vi "ConfigureDlg.vi"(8 "error in (no error)":errorcluster, 11 "PmuBase in":refnum<class "SensorBase.lvclass">) -> (0 "error out":errorcluster, 2 "Changed":bool, 3 "PmuBase out":refnum<class "SensorBase.lvclass">)   [LabVIEW 2014, in "SensorPlugins.lvlib" / "SensorBase.lvclass"]
uses:
  SensorBase.lvclass
panel:
  in  "btnDone":bool
  # "No configurable parameters for this Sensor plugin"
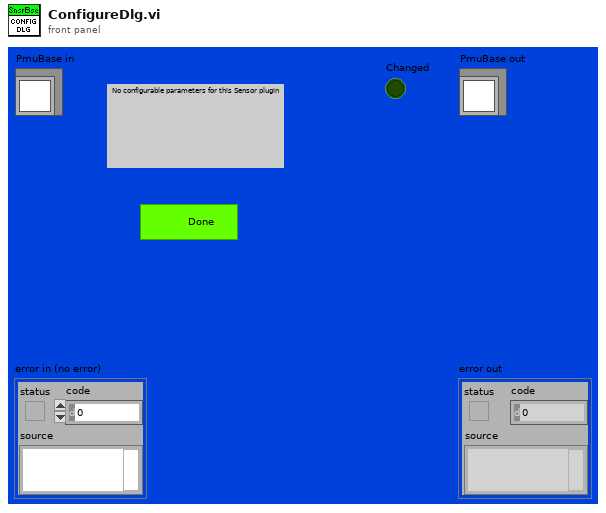
[diagram p1: front panel]
types:
  T1 = enum32{"Invalid", "Standard", "Closed", "Hidden", "Minimized", "Maximized"}
  T2 = enum32{"Invalid", "Default", "Floating", "Floating/Auto-Hide", "Modal"}
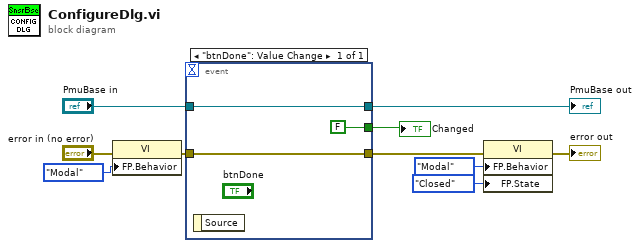
[diagram p0: block diagram]
diagram:
  n1 = property class="VI"(error in="error in (no error)", "FP.Behavior"=T2."Modal" ("Front Panel Window:Behavior")) -> (error out=w5:errorcluster)  [unwired: 1 in, 1 out]
  n2 = event shown="[0] \"btnDone\": Value Change" {
    selector: _ -> [_]
    dyn-events: _ -> [_]
    timeout: _ -> [_]
    tunnel: "PmuBase in" -> [w13]
    tunnel: [w13] -> w9
    tunnel: w5 -> [w12]
    tunnel: [w12] -> w7
    tunnel: [FALSE] -> w6
    event "btnDone": Value Change {
      n3 = event-data() -> ()  [unwired: 1 in, 1 out]
    }
  }
  "PmuBase out" <- w9
  "Changed" <- w6
  n4 = property class="VI"(error in=w7, "FP.Behavior"=T2."Modal" ("Front Panel Window:Behavior"), "FP.State"=T1."Closed" ("Front Panel Window:State")) -> (error out=→"error out":errorcluster)  [unwired: 1 in, 1 out]
